vi "Remove.vi"(8 "error in (no error)":errorcluster, 10 "BrowerComponentIDs(\"\")":string[](array[string]), 11 "reference in":refnum<class "BrowerComposite.lvclass">) -> (0 "error out":errorcluster, 3 "reference out":refnum<class "BrowerComposite.lvclass">)   [LabVIEW 2015, in "BrowerComposite.lvclass"]
uses:
  BrowerComposite.lvclass
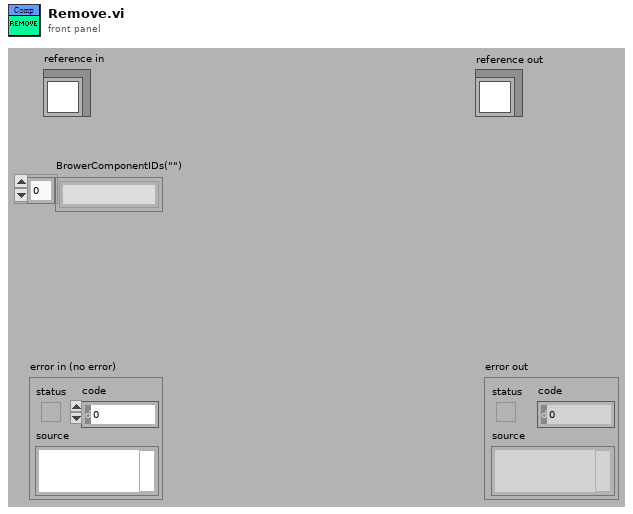
[diagram p1: front panel]
types:
  T1 = typedef "BrowerComposite.lvclass/ObjectAttributes.ctl" = cluster{"BrowerComponents":refnum<class "BrowerComponent.lvclass">[], "BrowerComponentIDs":string[], "Iterator":refnum<class "Iterator.lvclass">}
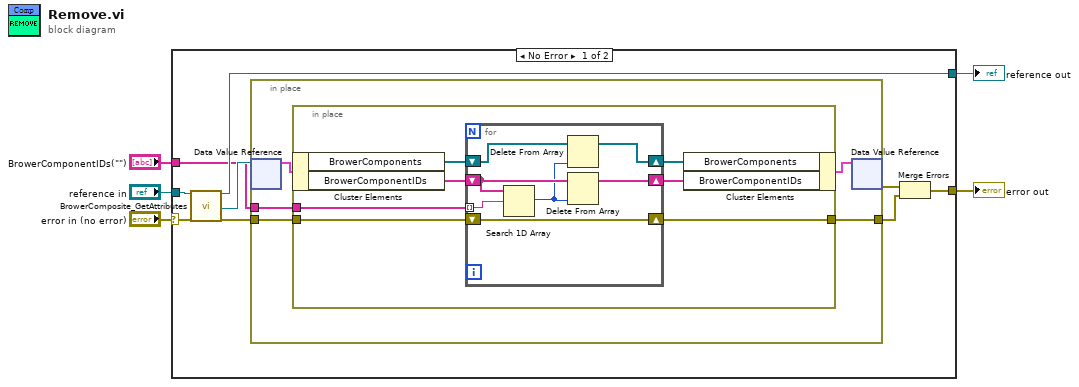
[diagram p0: block diagram]
diagram:
  n1 = case shown="No Error" "error in (no error)" {
    selector: "error in (no error)" -> [w13 w35]
    tunnel: [w11 w35] -> w4
    tunnel: [w10 w34] -> w2
    tunnel: "reference in" -> [w14 w34]
    tunnel: "BrowerComponentIDs(\"\")" -> [w8 _]
    frame No Error {
      n2 = call "BrowerComposite_GetAttributes.vi"("reference in"=w14, "error in (no error)"=w13) -> ("reference out"=w10:refnum<class "BrowerComposite.lvclass">, "DataRef"=w9:refnum<data-value>, "error out"=w7:errorcluster)  [unwired: 14 in, 1 out]
      n3 = in-place {
        in-place-border: w8 -> [w17]
        in-place-border: w7 -> [w16]
        in-place-border: [w15] -> w6
        n4 = in-place-dvr #1(w9) -> (w19:T1)  [unwired: 1 out]
        n5 = in-place {
          in-place-border: w17 -> [w26]
          in-place-border: w16 -> [w24]
          in-place-border: [w23] -> w15
          n6 = in-place-cluster #2(w19) -> ("BrowerComponents"=w25:refnum<class "BrowerComponent.lvclass">[], "BrowerComponentIDs"=w21:string[])
          n7 = for {
            tunnel: w26 -> [w32] mode=indexing
            shift-right: [w27] -> w22
            shift-left: w25 -> [w29]
            shift-right: [w33] -> w23
            shift-left: w24 -> [w33]
            shift-right: [w30] -> w20
            shift-left: w21 -> [w31]
            n8 = Search 1D Array(1D array=w31, element=w32) -> (index of element=w28:i32)  [unwired: 1 in]
            n9 = Delete From Array(array=w29, index=w28) -> (array with subset deleted=w27:refnum<class "BrowerComponent.lvclass">[])  [unwired: 1 in, 1 out]
            n10 = Delete From Array(array=w31, index=w28) -> (array with subset deleted=w30:string[])  [unwired: 1 in, 1 out]
          }
          n11 = in-place-cluster #2("BrowerComponents"=w22, "BrowerComponentIDs"=w20) -> (w18:T1)
        }
        n12 = in-place-dvr #1(w18) -> (w12:errorcluster)  [unwired: 1 out]
      }
      n13 = Merge Errors(w12, w6) -> (w11:errorcluster)
    }
    frame Error {
    }
  }
  "error out" <- w4
  "reference out" <- w2
